vi "init.vi"(6 "ID query?":bool, 7 "Reset?":bool, 8 "error in (no error)":errorcluster, 9 "connect timeout ms":i32=10000, 10 "port (502)":u16=502, 11 "address":string) -> (0 "error out":errorcluster, 2 "ID string":string, 3 "Modbus Master out":refnum<class "Modbus Master.lvclass">)   [LabVIEW 2018, in "ICP xET-7017.lvlib"]
uses:
  ICP xET-7017.lvlib
  <vilib>/NI/Modbus Library/API/Master/Modbus Master.lvclass
  <vilib>/NI/Modbus Library/API/Wrapper/Create TCP Master.vi
  <vilib>/NI/Modbus Library/API/Wrapper/API Main.lvlib
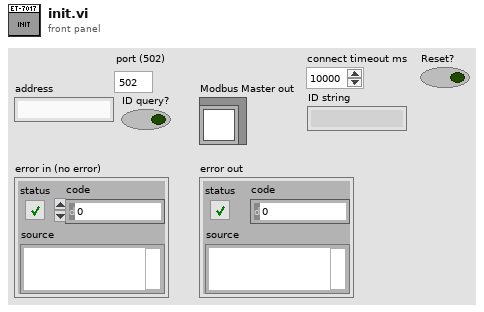
[diagram p1: front panel]
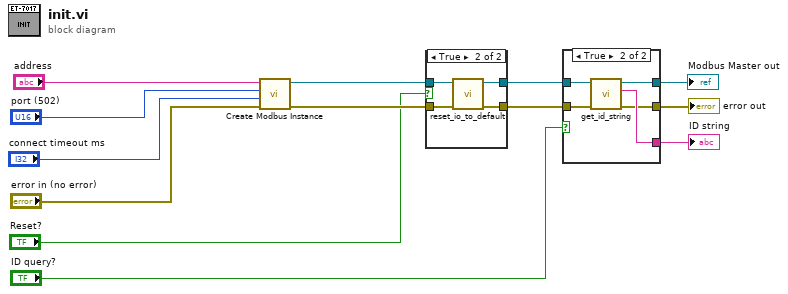
[diagram p0: block diagram]
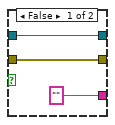
[diagram p3: hidden frame]
diagram:
  n1 = call-poly <vilib>:"Create Modbus Instance.vi"("error in"="error in (no error)", "connect timeout ms"="connect timeout ms", "port (502)"="port (502)", "address"="address") -> ("error out"=w3:errorcluster, "TCP master instance"=w2:refnum<class "Modbus Master.lvclass">)  [unwired: 6 in]
  n2 = case shown="True" "Reset?" {
    tunnel: w2 -> [w15 w19]
    tunnel: w3 -> [w14 w18]
    tunnel: [w14 w17] -> w4
    tunnel: [w15 w16] -> w5
    frame False {
    }
    frame True {
      n3 = call "reset_io_to_default.vi"("error in (no error)"=w18, "Modbus Master in"=w19) -> ("error out"=w17:errorcluster, "Modbus Master out"=w16:refnum<class "Modbus Master.lvclass">)  [unwired: 8 in]
    }
  }
  n4 = case shown="True" "ID query?" {
    tunnel: w5 -> [w22 w24]
    tunnel: [w22 w26] -> w9
    tunnel: w4 -> [w21 w23]
    tunnel: [w21 w25] -> w8
    tunnel: ["" w27] -> w6
    frame False {
    }
    frame True {
      n5 = call "get_id_string.vi"("error in (no error)"=w23, "Modbus Master in"=w24) -> ("error out"=w25:errorcluster, "String"=w27:string, "Modbus Master out"=w26:refnum<class "Modbus Master.lvclass">)  [unwired: 7 in]
    }
  }
  "error out" <- w8
  "Modbus Master out" <- w9
  "ID string" <- w6
